vi "Item_OnPopupMenu.vi"(11 "Object":T1) -> ()   [LabVIEW 2020, in "Triarc Project Provider.lvlib"]
uses:
  Triarc Project Provider.lvlib
  <resource>/Framework/Providers/API/ItemRef.ctl
  <resource>/Framework/Providers/API/mxLvMenuItem.ctl
panel:
  out "error out":errorcluster
  in  "error in":errorcluster
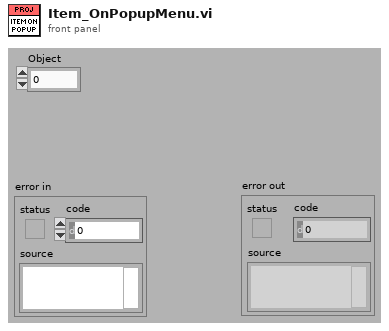
[diagram p1: front panel]
types:
  T1 = typedef "ItemRef.ctl" = u64
  T2 = typedef "mxLvMenuItem.ctl" = cluster{"Menu Name":string, "Description":string, "Icon File Name":path, "Menu Tag":string, "Enabled":bool, "Checked":bool, "Separator":bool, "Batchable":bool, "Weight":i32, "Batch Mode (Ignored if Not Batchable)":enum32{"Show If All Items Support Command", "Show If Any Items Support Command"}, "Menu Location":enum32{"<None>", "Project", "Project / Build Specifications", "Tools", "Tools / Source Control", "Tools / Real-Time Module", "Help"}, "Exclude From Getting Started Window Menu":bool}
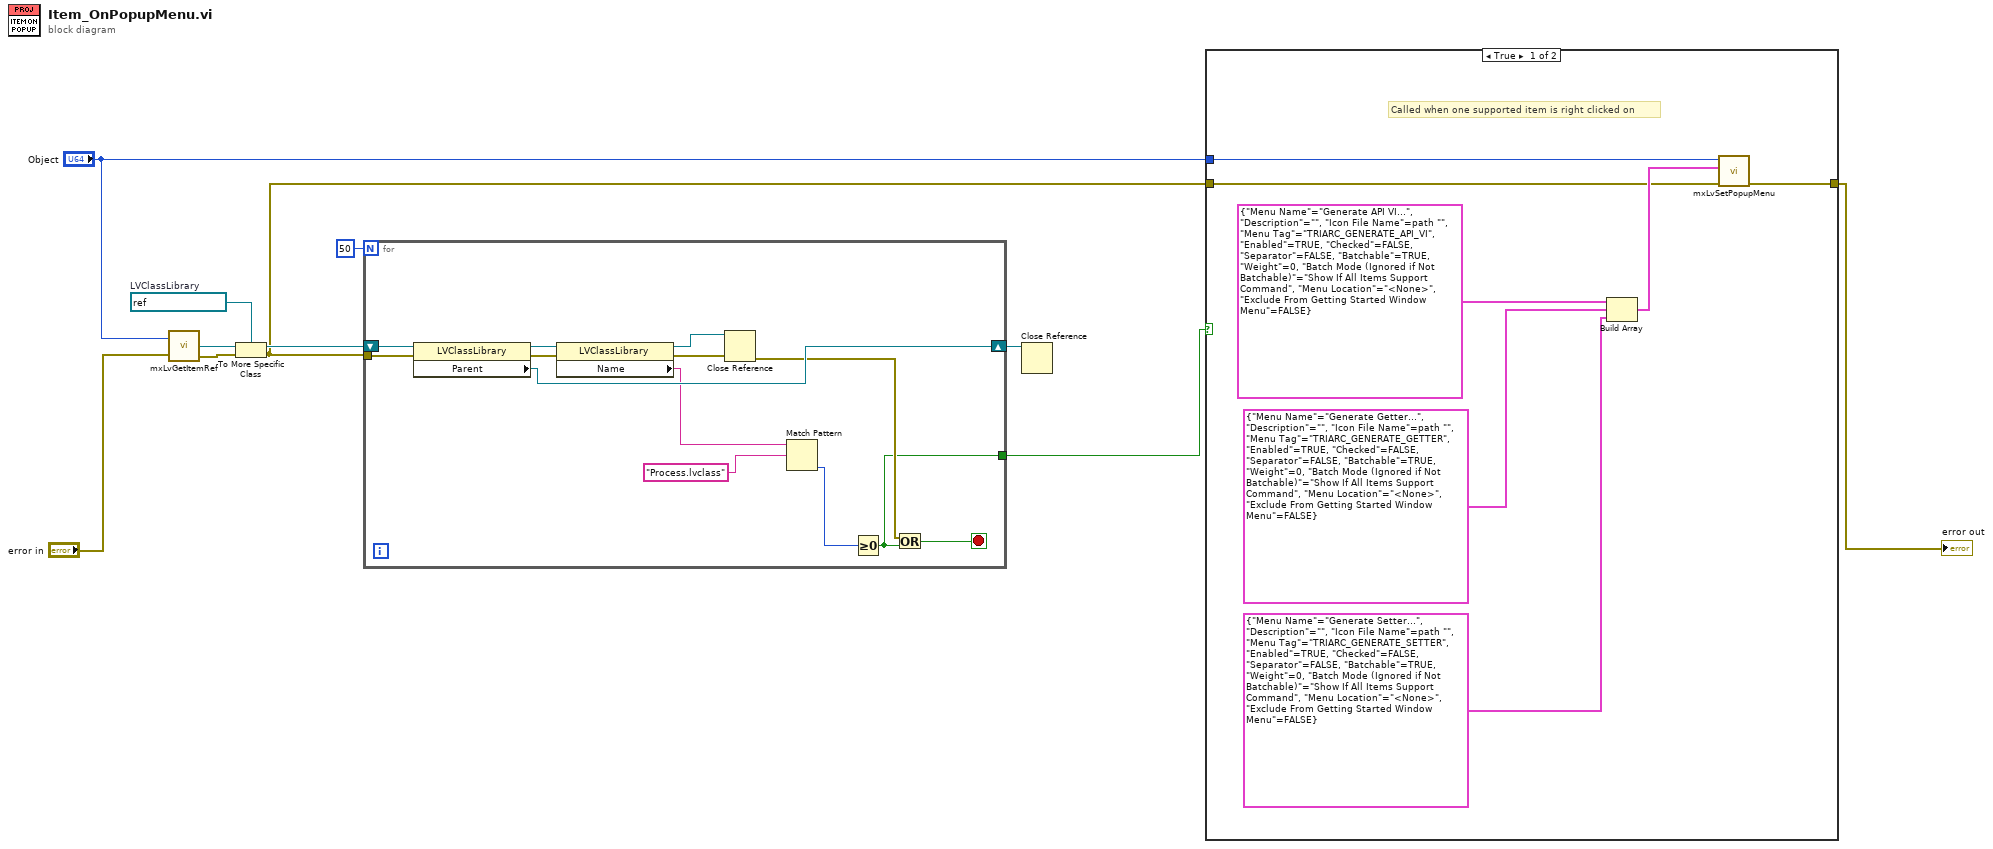
[diagram p0: block diagram]
diagram:
  w8 = refnum<vi> refnum  # LVClassLibrary
  n1 = call <resource>:"mxLvGetItemRef.vi"("Item"="Object", "error in"="error in") -> ("Item Refnum"=w10:refnum<vi>, "error out"=w7:errorcluster)  [unwired: 1 out]
  n2 = To More Specific Class(target class=w8, reference=w10, error in=w7) -> (specific class reference=w9:refnum<vi>, error out=w2:errorcluster)
  n3 = for {
    N: 50 -> [_]
    tunnel: w2 -> [w23]
    shift-right: [w22] -> w4
    shift-left: w9 -> [w24]
    tunnel: [w12] -> w1
    stop <- w14 stop-if-true
    n4 = property class="LVClassLibrary"(reference=w24, error in=w23) -> (reference out=w19:refnum<vi>, error out=w17:errorcluster, "Parent"=w22:refnum<vi>)
    n5 = property class="LVClassLibrary"(reference=w19, error in=w17) -> (reference out=w18:refnum<vi>, error out=w16:errorcluster, "Name"=w21:string)
    n6 = Close Reference(reference=w18, error in (no error)=w16) -> (error out=w20:errorcluster)
    n7 = Match Pattern(string=w21, regular expression="Process.lvclass" ("element")) -> (offset past match=w13:i32)  [unwired: 1 in, 3 out]
    n8 = Greater Or Equal To 0?(x=w13) -> (x >= 0?=w12:bool)
    n9 = Or(x=w20, y=w12) -> (x .or. y?=w14:bool)
  }
  n10 = Close Reference(reference=w4) -> ()  [unwired: 1 in, 1 out]
  n11 = case shown="True" w1 {
    tunnel: [w31 w32] -> w11
    tunnel: "Object" -> [w30 _]
    tunnel: w2 -> [w27 w32]
    frame True {
      # "Called when one supported item is right clicked on"
      n12 = Build Array(T2 {"Menu Name"="Generate API VI...", "Description"="", "Icon File Name"=path "", "Menu Tag"="TRIARC_GENERATE_API_VI", "Enabled"=TRUE, "Checked"=FALSE, "Separator"=FALSE, "Batchable"=TRUE, "Weight"=0, "Batch Mode (Ignored if Not Batchable)"=enum."Show If All Items Support Command", "Menu Location"=enum."<None>", "Exclude From Getting Started Window Menu"=FALSE} ("Menu Item"), T2 {"Menu Name"="Generate Getter...", "Description"="", "Icon File Name"=path "", "Menu Tag"="TRIARC_GENERATE_GETTER", "Enabled"=TRUE, "Checked"=FALSE, "Separator"=FALSE, "Batchable"=TRUE, "Weight"=0, "Batch Mode (Ignored if Not Batchable)"=enum."Show If All Items Support Command", "Menu Location"=enum."<None>", "Exclude From Getting Started Window Menu"=FALSE} ("Menu Item"), T2 {"Menu Name"="Generate Setter...", "Description"="", "Icon File Name"=path "", "Menu Tag"="TRIARC_GENERATE_SETTER", "Enabled"=TRUE, "Checked"=FALSE, "Separator"=FALSE, "Batchable"=TRUE, "Weight"=0, "Batch Mode (Ignored if Not Batchable)"=enum."Show If All Items Support Command", "Menu Location"=enum."<None>", "Exclude From Getting Started Window Menu"=FALSE} ("Menu Item")) -> (w29:T2[])
      n13 = call <resource>:"mxLvSetPopupMenu.vi"("error in"=w27, "Popup Menu Items"=w29, "Item"=w30) -> ("error out"=w31:errorcluster)  [unwired: 7 in, 1 out]
    }
    frame False {
    }
  }
  "error out" <- w11
